vi "SavePatientDateInfo_Palpation.vi"(8 "error in":errorcluster, 10 "side(left/right)":string, 11 "palpation":string) -> (0 "error out":errorcluster)   [LabVIEW 2013, in "main.lvlib"]
uses:
  main.lvlib
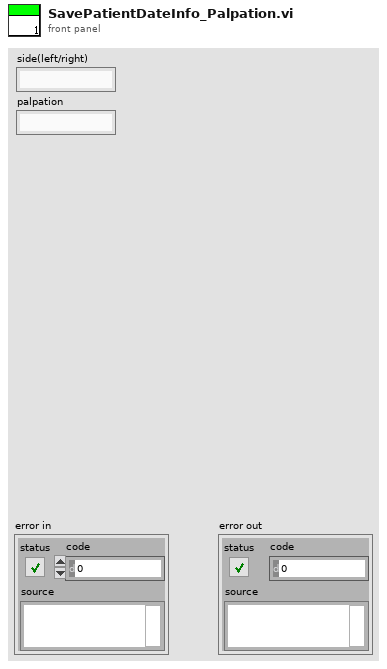
[diagram p1: front panel]
types:
  T1 = typedef "main.lvlib/date_specific_info.ctl" = cluster{"profile":cluster{"id":string, "name":string, "operator":string, "doctor":string, "comment":string}, "hospital":cluster{"name":string, "department":string, "address":string}, "palpation":cluster{"right":string, "left":string}, "Armpressure Right":cluster{"sys":dbl, "dia":dbl, "puls":dbl, "date":string, "time":string, "code":string, "serial":string, "temp":dbl, "activity":string}[], "Armpressure Left":cluster{"sys":dbl, "dia":dbl, "puls":dbl, "date":string, "time":string, "code":string, "serial":string, "temp":dbl, "activity":string}[]}
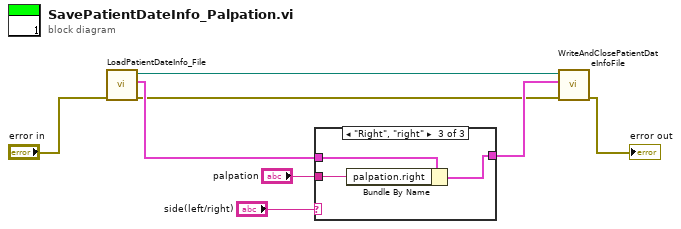
[diagram p0: block diagram]
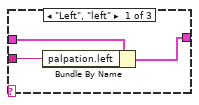
[diagram p2: hidden frame]
diagram:
  n1 = call "LoadPatientDateInfo_File.vi"("error in (no error)"="error in") -> ("error out"=w2:errorcluster, "date_specific_info"=w5:T1, "path"=w3:path)  [unwired: 8 in]
  n2 = case shown="\"Right\", \"right\"" "side(left/right)" {
    tunnel: [w9 w12 w13] -> w4
    tunnel: "palpation" -> [w11 _ w15]
    tunnel: w5 -> [w10 w12 w14]
    frame "Left", "left" {
      n3 = Bundle By Name(cluster=w10, "palpation.left"=w11) -> (w9:T1)
    }
    frame Default {
    }
    frame "Right", "right" {
      n4 = Bundle By Name(cluster=w14, "palpation.right"=w15) -> (w13:T1)
    }
  }
  n5 = call "WriteAndClosePatientDateInfoFile.vi"("error in (no error)"=w2, "date_specific_info"=w4, "file path (use dialog)"=w3) -> ("error out"=→"error out":errorcluster)  [unwired: 8 in]
